vi "Get Message Event Name.vi"(1 "Message":refnum<class "Message.lvclass">) -> (0 "Event Name":string)   [LabVIEW 2018]
uses:
  Classes/Message/Message.lvclass
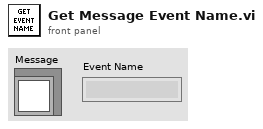
[diagram p1: front panel]
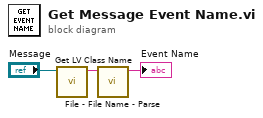
[diagram p0: block diagram]
diagram:
  n1 = call <vilib>:"Get LV Class Name.vi"("object"="Message") -> ("class name"=w2:string)  [unwired: 9 in, 1 out]
  n2 = call <userlib>:"File - File Name - Parse.vi"("File Name"=w2) -> ("Base Name"=→"Event Name":string)  [unwired: 8 in, 2 out]
